vi "Storage Thread.vi"(8 "error in (no error)":errorcluster, 9 "index":i32=3, 11 "Control Data":T1={"Queue Array"=[], "Queue Element"={"state"="", "data"=variant}, "System Event"=refnum, "System Event RefNum"=refnum, "Queue List"=[], "LPCA COM"="", "Rotating"=FALSE, "PrecorAI"="", "T_0 Index"=0, "Bar Graph X"=[], "Channels"=[], "Active Indicies"=[], "Active Channels"=[], "Sample Frequency"=0.0, "Ibrake Sweep"=[], "RPM Sweep"=[], "Load Sweep"=[], "Step Height Sweep"=[], "Range Sweep"=[], "A Counter"=0, "B Counter"=0, "C Counter"=0, "#A"=0, "#B"=0, "#C"=0, "Current RPM"=0.0, "Current Ibrake"=0, "Current Range"=0, "Current Step Height"=0, "Load Bank"=enum."OFF", "Cfg Cntrls"=[], "T_Monitor Indices"=[], "Thermal Limit"=0, "Thermal Resume"=0, "Timer Reset"=FALSE, "Stop Time"=0.0, "Autotest"=FALSE, "Pulsed RPM Capture"=FALSE, "Get Sample"=FALSE, "Last State"="", "Reset Timeout"=FALSE, "Ctrl Refs"={"Test Details"=refnum, "Save Config"=refnum, "Load Config"=refnum, "Path"=refnum, "Snapshot"=refnum, "SS#"=refnum, "Ibrake"=refnum, "RPM Target"=refnum, "Spin"=refnum, "Load Bank"=refnum, "Start Test"=refnum, "Pause Test"=refnum, "Load Sweep"=refnum, "RPM Sweep"=refnum, "Ibrake Sweep"=refnum, "Filters"=refnum, "Sample Frequency"=refnum, "Data Setup"=refnum, "Pause"=refnum, "Stop Time"=refnum, "S Period"=refnum, "Range"=refnum, "Step Height"=refnum, "Step Height Sweep"=refnum, "Range Sweep"=refnum, "Available Tests"=refnum, "RPM Graph"=refnum, "RPM Knob"=refnum, "FanMode"=refnum, "Fan Mode LED Array"=refnum, "Thermal Equilibrium"=refnum, "Data Display"=refnum, "LPCA Error"=refnum, "LPCA Ramp"=refnum, "LPCA Range"=refnum, "LPCA Resistance"=refnum, "Analyze Read"=refnum, "Console Select"=refnum, "Sub Panel"=refnum}, "Pulse Waveform"={"t0"=timestamp(0 s since 1904-01-01), "dt"=1.0, "Y"=[]}, "Snapshot"={"Test Details"="test", "Version"="test", "Date"=timestamp(3493915594.3018084 s since 1904-01-01), "Selected Test"="man", "Snapshot Number"=0, "Time"=timestamp(3493915602.7292905 s since 1904-01-01), "Ibrake Setpoint"="1", "RPM Setpoint"="20", "Range Setpoint"="", "Step Height Setpoint"="", "Load Bank Setpoint"="15", "Measurement Headers"="a,b,c,1,2,3", "Measurements"="1,2,3,4,5,6,7,8", "A"=0, "B"=0, "C"=0, "Raw Data"=[], "Available Tests"=enum."Manual", "Ibrake List"="", "RPM List"="", "Load Bank List"="", "Range List"="", "Step Height List"="", "FanMode Setpoint"=enum."Auto"}, "Sample Period"=0.0, "OverTemp"=FALSE, "Available Tests"=enum."Manual", "FanMode"=enum."Auto", "Fan Mode LED Array"=[FALSE, TRUE, FALSE], "Thermal\nEquilibrium "=FALSE, "Equilibrium Stop"=FALSE, "AvgDegChg"=[]} {"Snapshot"."Time" format="%<%H:%M:%S>T"; "Snapshot"."Date" format="%<%m/%d/%Y>T"}) -> ()   [LabVIEW 2017]
uses:
  Controls/Test TypeDef.ctl
  Code Library/Queue References Array.ctl
  Code Library/Queue Element.ctl
  Controls/Load Bank.ctl
  Controls/Available Tests.ctl
  Console Sim/Controls/Console Select.ctl
  Controls/Snapshot Typedef.ctl
  Controls/FanMode.ctl
  <vilib>/Waveform/WDTFileIO.llb/Export Waveforms To Spreadsheet File (1D).vi
  <vilib>/Utility/file.llb/Write To Spreadsheet File (string).vi
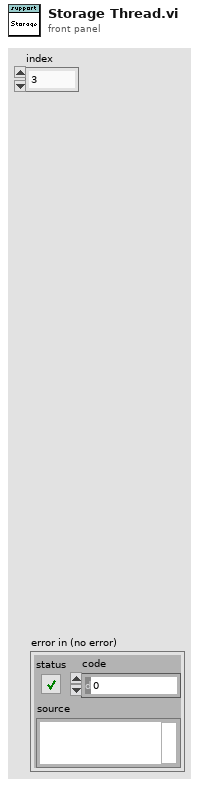
[diagram p1: front panel]
types:
  T1 = typedef "Test TypeDef.ctl" = cluster{"Queue Array":T2, "Queue Element":T3, "System Event":refnum<user-event>, "System Event RefNum":refnum<event-registration>, "Queue List":string[], "LPCA COM":refnum<visa-resource-name>, "Rotating":bool, "PrecorAI":refnum<k21>, "T_0 Index":i32, "Bar Graph X":i32[], "Channels":string[], "Active Indicies":i32[], "Active Channels":string[][], "Sample Frequency":dbl, "Ibrake Sweep":string[], "RPM Sweep":string[], "Load Sweep":string[], "Step Height Sweep":string[], "Range Sweep":string[], "A Counter":i32, "B Counter":i32, "C Counter":i32, "#A":i32, "#B":i32, "#C":i32, "Current RPM":dbl, "Current Ibrake":u32, "Current Range":u32, "Current Step Height":u32, "Load Bank":T4, "Cfg Cntrls":refnum<vi>[], "T_Monitor Indices":i32[], "Thermal Limit":i32, "Thermal Resume":i32, "Timer Reset":bool, "Stop Time":dbl, "Autotest":bool, "Pulsed RPM Capture":bool, "Get Sample":bool, "Last State":string, "Reset Timeout":bool, "Ctrl Refs":cluster{"Test Details":refnum<vi>, "Save Config":refnum<vi>, "Load Config":refnum<vi>, "Path":refnum<vi>, "Snapshot":refnum<vi>, "SS#":refnum<vi>, "Ibrake":refnum<vi>, "RPM Target":refnum<vi>, "Spin":refnum<vi>, "Load Bank":refnum<vi>, "Start Test":refnum<vi>, "Pause Test":refnum<vi>, "Load Sweep":refnum<vi>, "RPM Sweep":refnum<vi>, "Ibrake Sweep":refnum<vi>, "Filters":refnum<vi>, "Sample Frequency":refnum<vi>, "Data Setup":refnum<vi>, "Pause":refnum<vi>, "Stop Time":refnum<vi>, "S Period":refnum<vi>, "Range":refnum<vi>, "Step Height":refnum<vi>, "Step Height Sweep":refnum<vi>, "Range Sweep":refnum<vi>, "Available Tests":refnum<vi>, "RPM Graph":refnum<vi>, "RPM Knob":refnum<vi>, "FanMode":refnum<vi>, "Fan Mode LED Array":refnum<vi>, "Thermal Equilibrium":refnum<vi>, "Data Display":refnum<vi>, "LPCA Error":refnum<vi>, "LPCA Ramp":refnum<vi>, "LPCA Range":refnum<vi>, "LPCA Resistance":refnum<vi>, "Analyze Read":refnum<vi>, "Console Select":refnum<vi>, "Sub Panel":refnum<vi>}, "Pulse Waveform":waveform(dbl), "Snapshot":T5, "Sample Period":dbl, "OverTemp":bool, "Available Tests":T6, "FanMode":T7, "Fan Mode LED Array":bool[], "Thermal\nEquilibrium ":bool, "Equilibrium Stop":bool, "AvgDegChg":dbl[]}
  T2 = typedef "Queue References Array.ctl" = refnum<queue>[]
  T3 = typedef "Queue Element.ctl" = cluster{"state":string, "data":variant}
  T4 = typedef "Load Bank.ctl" = enum16{"OFF", "50", "25", "16.7", "12.5", "10.0", "8.3", "7.1", "6.3", "5.6", "5.0", "4.5", "4.2", "3.8", "3.6", "3.3", "3.1"}
  T5 = typedef "Snapshot Typedef.ctl" = cluster{"Test Details":string, "Version":string, "Date":timestamp, "Selected Test":string, "Snapshot Number":u16, "Time":timestamp, "Ibrake Setpoint":string, "RPM Setpoint":string, "Range Setpoint":string, "Step Height Setpoint":string, "Load Bank Setpoint":string, "Measurement Headers":string, "Measurements":string, "A":i32, "B":i32, "C":i32, "Raw Data":string[][], "Available Tests":T6, "Ibrake List":string, "RPM List":string, "Load Bank List":string, "Range List":string, "Step Height List":string, "FanMode Setpoint":T7}
  T6 = typedef "Available Tests.ctl" = enum16{"Manual", "EFX Brake Torque", "Generator Torque", "EFX Brake Thermal", "Generator Thermal", "Pulsed RPM", "AMT Brake Torque", "Bike Brake Torque", "AMT Brake Thermal", "Bike Brake Thermal"}
  T7 = typedef "FanMode.ctl" = enum16{"On", "Off", "Auto"}
  T8 = cluster{"task in":refnum<k21>, "MulticolumnListbox in":refnum<vi>, "Snapshot":T5, bool, "Torque":dbl, "RPM":dbl}
  T9 = cluster{"Control Data":T1, "Current File":path, "New File":bool, "Snapshot":u16, "Last State":string}
  T10 = enum16{"open", "replace", "create", "open or create", "replace or create", "replace or create with confirmation"}
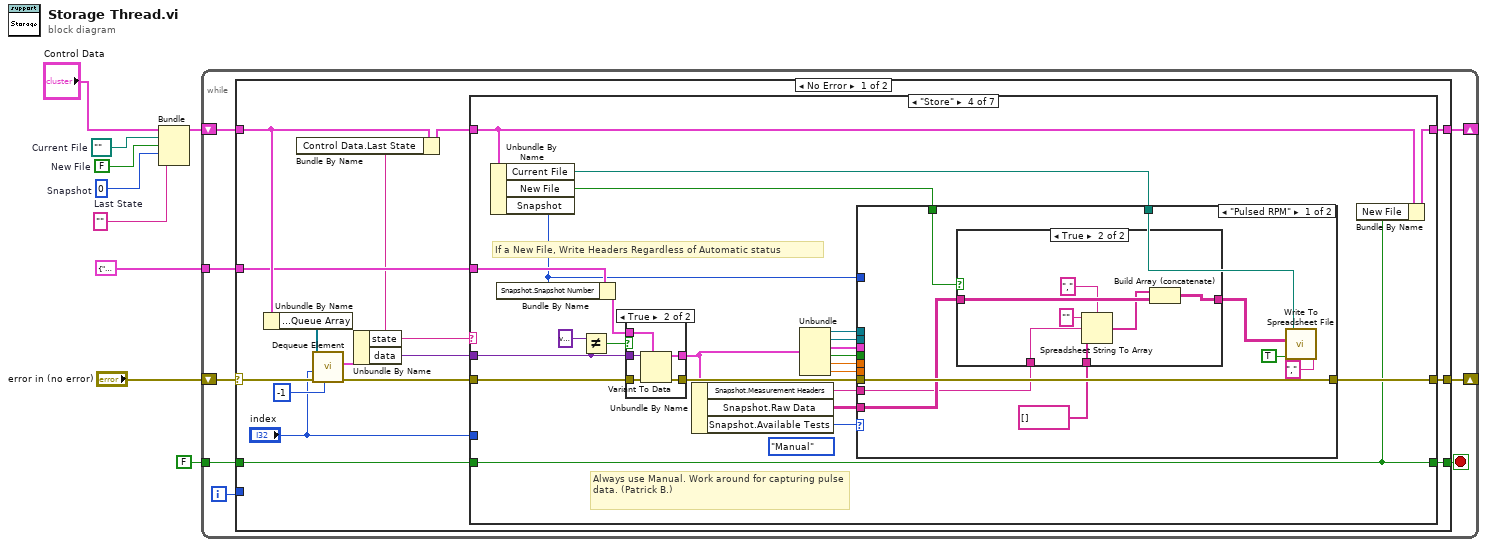
[diagram p0: block diagram]
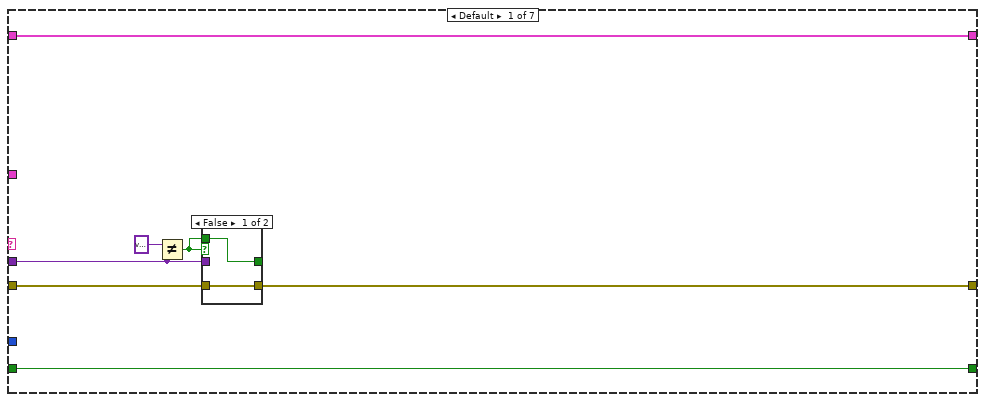
[diagram p2: hidden frame]
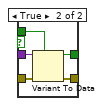
[diagram p3: hidden frame]
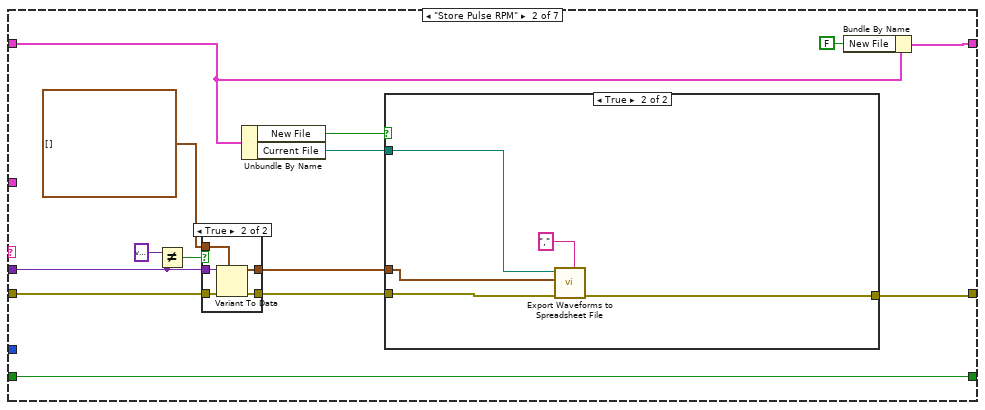
[diagram p4: hidden frame]
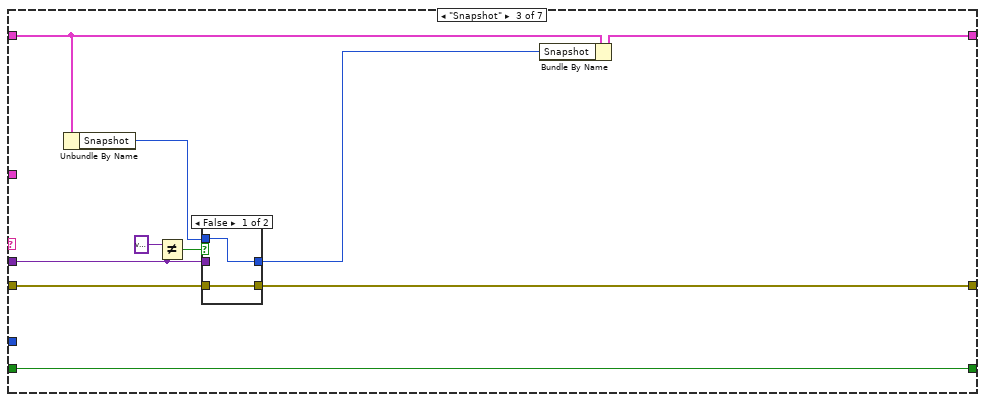
[diagram p7: hidden frame]
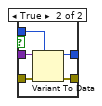
[diagram p8: hidden frame]
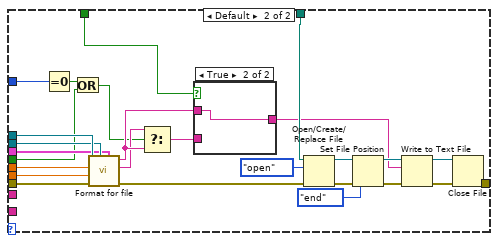
[diagram p10: hidden frame]
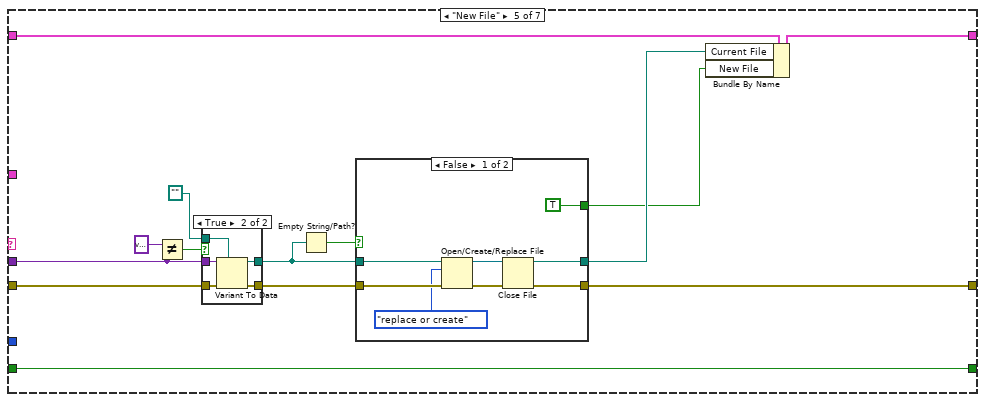
[diagram p13: hidden frame]
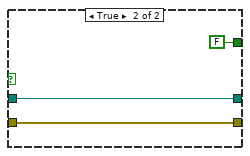
[diagram p14: hidden frame]
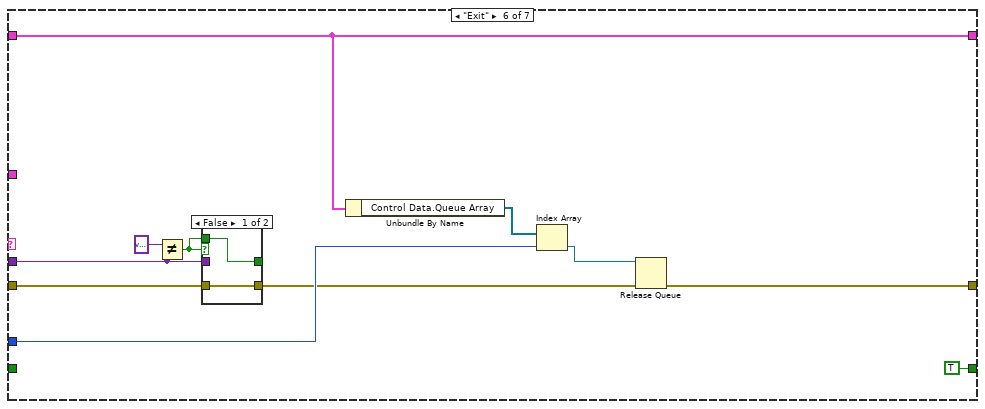
[diagram p16: hidden frame]
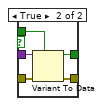
[diagram p17: hidden frame]
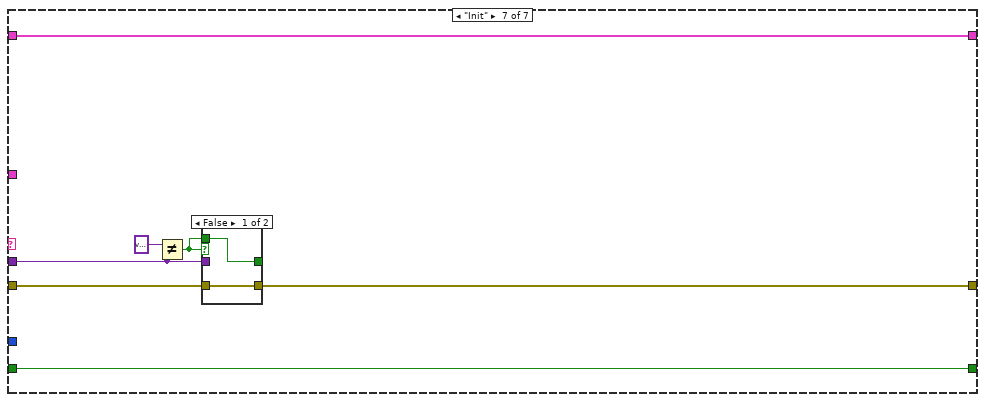
[diagram p18: hidden frame]
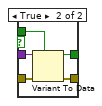
[diagram p19: hidden frame]
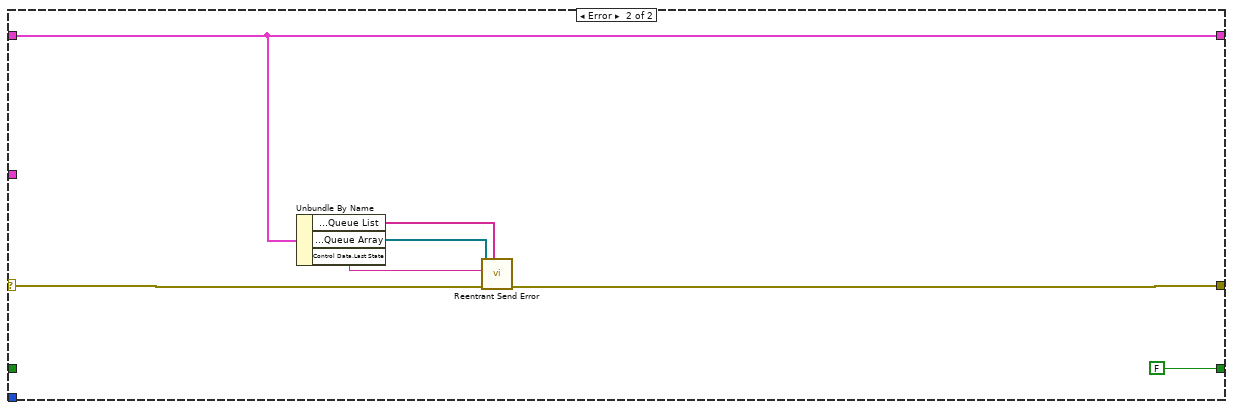
[diagram p20: hidden frame]
diagram:
  w3 = ""  # Last State
  w4 = u16 0  # Snapshot
  w5 = FALSE  # New File
  w6 = path ""  # Current File
  n1 = Bundle("Control Data"="Control Data", "Current File"=w6, "New File"=w5, "Snapshot"=w4, "Last State"=w3) -> (w7:T9)  [unwired: 1 in]
  n2 = while {
    shift-right: [w12] -> _
    shift-left: w7 -> [w17]
    tunnel: FALSE ("Boolean") -> [w14]
    shift-right: [w15] -> _
    shift-left: "error in (no error)" -> [w16]
    tunnel: T8 {"task in"="", "MulticolumnListbox in"=refnum, "Snapshot"={"Test Details"="", "Version"="test", "Date"=timestamp(0 s since 1904-01-01), "Selected Test"="", "Snapshot Number"=0, "Time"=timestamp(0 s since 1904-01-01), "Ibrake Setpoint"="", "RPM Setpoint"="", "Range Setpoint"="", "Step Height Setpoint"="", "Load Bank Setpoint"="", "Measurement Headers"="", "Measurements"="", "A"=0, "B"=0, "C"=0, "Raw Data"=[], "Available Tests"=enum."Manual", "Ibrake List"="", "RPM List"="", "Load Bank List"="", "Range List"="", "Step Height List"="", "FanMode Setpoint"=enum."Auto"}, FALSE, "Torque"=0.0, "RPM"=0.0} ("snapshot") -> [w11]
    i -> [w10]
    stop <- w13 stop-if-true
    n3 = case shown="No Error" w16 {
      selector: w16 -> [w30 w235]
      tunnel: w17 -> [w23 w236]
      tunnel: [w28 w234] -> w15
      tunnel: w14 -> [w27 _]
      tunnel: [w26 FALSE ("Boolean")] -> w13
      tunnel: [w24 w236] -> w12
      tunnel: w11 -> [w21 _]
      tunnel: w10 -> [_ _]
      frame No Error {
        n4 = Unbundle By Name(w23) -> ("Control Data.Queue Array"=w32:T2)
        n5 = call "Dequeue Element.vi"("timeout in ms (-1)"=-1, "error in (no error)"=w30, "index"="index", "Queue Array"=w32) -> ("error out"=w29:errorcluster, "Queue Element"=w18:T3)  [unwired: 5 in, 1 out]
        n6 = Unbundle By Name(w18) -> ("state"=w19:string, "data"=w25:variant)
        n7 = Bundle By Name(cluster=w23, "Control Data.Last State"=w19) -> (w20:T9)
        n8 = case shown="\"Store\"" w19 {
          tunnel: w29 -> [w37 w59 w82 w114 w178 w209 w222]
          tunnel: [w36 w47 w74 w108 w171 w199 w218] -> w28
          tunnel: w27 -> [w39 w60 w83 w104 w180 _ w223]
          tunnel: [w39 w60 w83 w104 w180 TRUE ("Boolean") w223] -> w26
          tunnel: w25 -> [w34 w57 w80 w112 w175 w207 w220]
          tunnel: [w38 w54 w76 w105 w170 w204 w217] -> w24
          tunnel: w20 -> [w38 w53 w78 w106 w179 w204 w217]
          tunnel: "index" -> [_ _ _ _ _ w202 _]
          tunnel: w21 -> [_ _ _ w103 _ _ _]
          frame Default {
            n9 = Not Equal?(x=variant, y=w34) -> (x != y?=w33:bool)
            n10 = case shown="False" w33 {
              tunnel: w37 -> [w41 w46]
              tunnel: [w41 w45] -> w36
              tunnel: w34 -> [_ w44]
              tunnel: [w40 w43] -> _
              tunnel: w33 -> [w40 w42]
              frame False {
              }
              frame True {
                n11 = Variant To Data(error in=w46, type=w42, Variant=w44) -> (data=w43:bool, error out=w45:errorcluster)
              }
            }
          }
          frame "Store Pulse RPM" {
            n12 = Not Equal?(x=variant, y=w57) -> (x != y?=w56:bool)
            n13 = case shown="True" w56 {
              tunnel: w59 -> [w68 w73]
              tunnel: [w68 w72] -> w49
              tunnel: w57 -> [_ w71]
              tunnel: [w67 w70] -> w48
              tunnel: waveform(dbl)[] [] ("Pulse RPM Data") -> [w67 w69]
              frame False {
              }
              frame True {
                n14 = Variant To Data(error in=w73, type=w69, Variant=w71) -> (data=w70:waveform(dbl)[], error out=w72:errorcluster)
              }
            }
            n15 = Unbundle By Name(w53) -> ("New File"=w51:bool, "Current File"=w50:path)
            n16 = case shown="True" w51 {
              tunnel: w50 -> [_ w64]
              tunnel: w49 -> [w61 w65]
              tunnel: w48 -> [_ w66]
              tunnel: [w61 w63] -> w47
              frame False {
              }
              frame True {
                n17 = call-poly <vilib>:"Export Waveforms to Spreadsheet File.vi"("delimiter (Tab)"=",", "error in (no error)"=w65, "waveforms"=w66, "file path (dialog if empty)"=w64) -> ("error out"=w63:errorcluster)  [unwired: 6 in, 1 out]
              }
            }
            n18 = Bundle By Name(cluster=w53, "New File"=FALSE) -> (w54:T9)
          }
          frame "Snapshot" {
            n19 = Unbundle By Name(w78) -> ("Snapshot"=w77:u16)
            n20 = Not Equal?(x=variant, y=w80) -> (x != y?=w79:bool)
            n21 = case shown="False" w79 {
              tunnel: w82 -> [w85 w90]
              tunnel: [w85 w89] -> w74
              tunnel: w80 -> [_ w88]
              tunnel: [w84 w87] -> w75
              tunnel: w77 -> [w84 w86]
              frame False {
              }
              frame True {
                n22 = Variant To Data(error in=w90, type=w86, Variant=w88) -> (data=w87:u16, error out=w89:errorcluster)
              }
            }
            n23 = Bundle By Name(cluster=w78, "Snapshot"=w75) -> (w76:T9)
          }
          frame "Store" {
            (unwired) Available_Tests."Manual" ("Available Tests")
            # "Always use Manual. Work around for capturing pulse data. (Patrick B.)"
            # "If a New File, Write Headers Regardless of Automatic status"
            n24 = Unbundle By Name(w106) -> ("Current File"=w109:path, "New File"=w107:bool, "Snapshot"=w101:u16)
            n25 = Bundle By Name(cluster=w103, "Snapshot.Snapshot Number"=w101) -> (w102:T8)
            n26 = Not Equal?(x=variant, y=w112) -> (x != y?=w111:bool)
            n27 = case shown="True" w111 {
              tunnel: w114 -> [w161 w166]
              tunnel: [w161 w165] -> w110
              tunnel: w112 -> [_ w164]
              tunnel: [w160 w163] -> w99
              tunnel: w102 -> [w160 w162]
              frame False {
              }
              frame True {
                n28 = Variant To Data(error in=w166, type=w162, Variant=w164) -> (data=w163:T8, error out=w165:errorcluster)
              }
            }
            n29 = Unbundle By Name(w99) -> ("Snapshot.Measurement Headers"=w92:string, "Snapshot.Raw Data"=w100:string[][], "Snapshot.Available Tests"=w91:T6)
            n30 = Unbundle(w99) -> ("task in"=w98:refnum<k21>, "MulticolumnListbox in"=w97:refnum<vi>, "Snapshot"=w96:T5, w95:bool, "Torque"=w94:dbl, "RPM"=w93:dbl)
            n31 = case shown="\"Pulsed RPM\"" w91 {
              tunnel: w110 -> [w123 w157]
              tunnel: w109 -> [w122 w150]
              tunnel: [w123 w148] -> w108
              tunnel: w107 -> [w120 w145]
              tunnel: w101 -> [_ w139]
              tunnel: w100 -> [w119 _]
              tunnel: w98 -> [_ w137]
              tunnel: w97 -> [_ w136]
              tunnel: w96 -> [_ w135]
              tunnel: w95 -> [_ w134]
              tunnel: w94 -> [_ w133]
              tunnel: w93 -> [_ w132]
              tunnel: w92 -> [w116 _]
              frame "Pulsed RPM" {
                n32 = case shown="True" w120 {
                  tunnel: w119 -> [w124 w131]
                  tunnel: [w124 w130] -> w118
                  tunnel: w116 -> [_ w129]
                  tunnel: string[] [] ("Raw Data") -> [_ w128]
                  frame False {
                  }
                  frame True {
                    n33 = Spreadsheet String To Array(delimiter (Tab)=",", format string="", spreadsheet string=w129, array type (2D Dbl)=w128) -> (array=w127:string[])
                    n34 = Build Array (concatenate)(w127, w131) -> (w130:string[][])
                  }
                }
                n35 = call-poly <vilib>:"Write To Spreadsheet File.vi"("delimiter (\\t)"="," ("delimiter (\\t)"), "append to file? (new file:F)"=TRUE, "2D data"=w118, "file path (dialog if empty)"=w122) -> ()  [unwired: 4 in, 1 out]
              }
              frame Default {
                n36 = Equal To 0?(x=w139) -> (x = 0?=w138:bool)
                n37 = Or(x=w138, y=w134) -> (x .or. y?=w140:bool)
                n38 = call "Format for file.vi"("Snapshot"=w135, "Data Setup"=w136, "error in (no error)"=w157, "RPM"=w132, "Torque"=w133, "DAQmx Task Name"=w137) -> ("error out"=w149:errorcluster, "Measurements"=w143:string, "Headers and Measurements"=w144:string)  [unwired: 3 in]
                n39 = Select(t=w143, s=w140, f=w144) -> (s? t:f=w141:string)
                n40 = case shown="True" w145 {
                  tunnel: w144 -> [_ w159]
                  tunnel: [w158 w159] -> w142
                  tunnel: w141 -> [w158 _]
                  frame False {
                  }
                  frame True {
                  }
                }
                n41 = Open/Create/Replace File(file path (use dialog)=w150, error in=w149, operation (0:open)=T10."open") -> (refnum out=w155:refnum<file>, error out=w156:errorcluster)  [unwired: 3 in, 1 out]
                n42 = Set File Position(refnum=w155, from (0:start)=enum16{"start", "end", "current"}."end", error in=w156) -> (refnum out=w151:refnum<file>, error out=w154:errorcluster)  [unwired: 1 in]
                n43 = Write to Text File(file (use dialog)=w151, text=w142, error in=w154) -> (refnum out=w152:refnum<file>, error out=w153:errorcluster)  [unwired: 1 in, 1 out]
                n44 = Close File(refnum=w152, error in=w153) -> (error out=w148:errorcluster)  [unwired: 1 out]
              }
            }
            n45 = Bundle By Name(cluster=w106, "New File"=w104) -> (w105:T9)
          }
          frame "New File" {
            n46 = Not Equal?(x=variant, y=w175) -> (x != y?=w174:bool)
            n47 = case shown="True" w174 {
              tunnel: w178 -> [w193 w198]
              tunnel: [w193 w197] -> w177
              tunnel: w175 -> [_ w196]
              tunnel: [w192 w195] -> w172
              tunnel: path "" -> [w192 w194]
              frame False {
              }
              frame True {
                n48 = Variant To Data(error in=w198, type=w194, Variant=w196) -> (data=w195:path, error out=w197:errorcluster)
              }
            }
            n49 = Empty String/Path?(string/path=w172) -> (empty?=w168:bool)
            n50 = case shown="False" w168 {
              tunnel: w177 -> [w188 w191]
              tunnel: w172 -> [w186 w190]
              tunnel: [w184 w191] -> w171
              tunnel: [w182 w190] -> w169
              tunnel: [TRUE FALSE] -> w167
              frame False {
                n51 = Open/Create/Replace File(file path (use dialog)=w186, error in=w188, operation (0:open)=T10."replace or create") -> (refnum out=w183:refnum<file>, error out=w187:errorcluster)  [unwired: 3 in, 1 out]
                n52 = Close File(refnum=w183, error in=w187) -> (path=w182:path, error out=w184:errorcluster)
              }
              frame True {
              }
            }
            n53 = Bundle By Name(cluster=w179, "Current File"=w169, "New File"=w167) -> (w170:T9)
          }
          frame "Exit" {
            n54 = Not Equal?(x=variant, y=w207) -> (x != y?=w206:bool)
            n55 = case shown="False" w206 {
              tunnel: w209 -> [w211 w216]
              tunnel: [w211 w215] -> w200
              tunnel: w207 -> [_ w214]
              tunnel: [w210 w213] -> _
              tunnel: w206 -> [w210 w212]
              frame False {
              }
              frame True {
                n56 = Variant To Data(error in=w216, type=w212, Variant=w214) -> (data=w213:bool, error out=w215:errorcluster)
              }
            }
            n57 = Unbundle By Name(w204) -> ("Control Data.Queue Array"=w203:T2)
            n58 = Index Array(array=w203, index=w202) -> (element=w201:refnum<queue>)
            n59 = Release Queue(queue=w201, error in (no error)=w200) -> (error out=w199:errorcluster)  [unwired: 1 in, 2 out]
          }
          frame "Init" {
            n60 = Not Equal?(x=variant, y=w220) -> (x != y?=w219:bool)
            n61 = case shown="False" w219 {
              tunnel: w222 -> [w225 w230]
              tunnel: [w225 w229] -> w218
              tunnel: w220 -> [_ w228]
              tunnel: [w224 w227] -> _
              tunnel: w219 -> [w224 w226]
              frame False {
              }
              frame True {
                n62 = Variant To Data(error in=w230, type=w226, Variant=w228) -> (data=w227:bool, error out=w229:errorcluster)
              }
            }
          }
        }
      }
      frame Error {
        n63 = Unbundle By Name(w236) -> ("Control Data.Queue List"=w232:string[], "Control Data.Queue Array"=w233:T2, "Control Data.Last State"=w237:string)
        n64 = call "Reentrant Send Error.vi"("Queue Names"=w232, "error in (no error)"=w235, "Last State"=w237, "Queues"=w233) -> ("error out"=w234:errorcluster)  [unwired: 7 in]
      }
    }
  }
